vi "ARGBImageSize.vi"(8 "error in (no error)":errorcluster, 11 "ARGB Image":refnum<data-value>) -> (0 "error out":errorcluster, 2 "Image Size":T1, 3 "ARGB Image (duplicate)":refnum<data-value>)   [LabVIEW 2020, in "g_ar_toolkit.image.lvlib"]
uses:
  g_ar_toolkit.image.lvlib
  g_ar_toolkit.common/Image Size (Integer).ctl
  69a1505b-b287-44ed-9ef9-f10ed7b260f4.vi
  g_ar_toolkit.common/g_ar_toolkit.common.lvlib
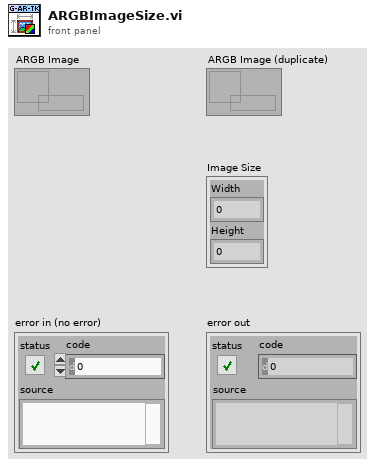
[diagram p1: front panel]
types:
  T1 = typedef "g_ar_toolkit.common.lvlib/Image Size (Integer).ctl" = cluster{"Width":u16, "Height":u16}
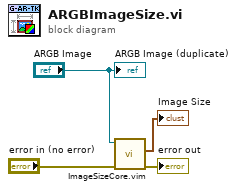
[diagram p0: block diagram]
diagram:
  n1 = call "ImageSizeCore.vim"("error in (no error)"="error in (no error)", "Image"="ARGB Image") -> ("error out"=→"error out":errorcluster, "Image Size"=→"Image Size":T1)  [unwired: 8 in]
  "ARGB Image (duplicate)" <- "ARGB Image"
